vi "XY Galvo Generator Underscan.v2.Filter.vi"(3 "Microscope Settings in":T1={"Mode"=enum."X", "Slit"={"Scanning Mode"=0.0, "Slit Width /%"=0.0}, "Colour Channel"=enum."3", "Colour"=[], "Focus Offset /um"=0.0, "Exposure/ms"=0.0, "Piezo Position /um"=0.0, "ROI"={"X"={"Start /px"=0.0, "Step /px"=0.0, "Range /px"=0.0}, "Y"={"Start /px"=0.0, "Step /px"=0.0, "Range /px"=0.0}, "Z "={"Start /um"=0.0, "Step/um"=0.0, "Range /um"=0.0}, "T "={"Start /s"=0.0, "Step /s"=1.0, "Range /s"=100.0}}, "Samples per millisecond"=0.0, "Relax/ms"=0.0, "Readout Direction"=0.0, "Trigger Source"=0.0, "Camera Delay /ms"=0.0, "Under Scan /ms"=0.0, "Slit Delay"=100.0, "Waveforms"={"Analogue Out"=[{"t0"=timestamp(0 s since 1904-01-01), "dt"=1.0, "Y"=[]}, {"t0"=timestamp(0 s since 1904-01-01), "dt"=1.0, "Y"=[]}, {"t0"=timestamp(0 s since 1904-01-01), "dt"=1.0, "Y"=[]}], "Digital Out"=[{"t0"=timestamp(0 s since 1904-01-01), "dt"=0.0, "Y"={"transitions"=[], "data"=[]}}, {"t0"=timestamp(0 s since 1904-01-01), "dt"=0.0, "Y"={"transitions"=[], "data"=[]}}, {"t0"=timestamp(0 s since 1904-01-01), "dt"=0.0, "Y"={"transitions"=[], "data"=[]}}]}} {"Focus Offset /um" min=0.0 max=10.0 step=0.05 scale=-2.0..2.0 scale format="%.2f"; "ROI"."T"."Range /s" min=0.0 max=10.0 step=0.05; "ROI"."T"."Step /s" min=0.0 max=10.0 step=0.05; "ROI"."T"."Start /s" min=0.0 max=10.0 step=0.05; "ROI"."X"."Range /px" min=0.0 max=10.0 step=0.05; "ROI"."X"."Step /px" min=0.0 max=10.0 step=0.05; "ROI"."X"."Start /px" min=0.0 max=10.0 step=0.05; "ROI"."Y"."Range /px" min=0.0 max=10.0 step=0.05; "ROI"."Y"."Step /px" min=0.0 max=10.0 step=0.05; "ROI"."Y"."Start /px" min=0.0 max=10.0 step=0.05; "ROI"."Z"."Range /um" min=0.0 max=10.0 step=0.05; "ROI"."Z"."Step/um" min=0.0 max=10.0 step=0.05; "ROI"."Z"."Start /um" min=0.0 max=10.0 step=0.05; "Colour"."Colour"."Filter" items=["Empty"=1, ""=2, ""=3, "561"=4, ""=5, "488"=6]; "Camera Delay /ms" min=0.0 max=10.0 step=0.05; "Trigger Source" items=["Internal"=1.0, "External"=2.0]; "Readout Direction" items=["Internal"=1.0, "External"=2.0]; "Slit"."Scanning Mode" items=["Full Frame"=1.0, "Slit Scanning"=12.0]; "Piezo Position /um" min=0.0 max=10.0 step=0.05; "Exposure/ms" min=0.0 max=10.0 step=0.05; "Samples per millisecond" min=1.0 max=2.0 step=1.0}) -> (0 "Piezo":dbl[](graph))   [LabVIEW 2016]
uses:
  controls/Microscope Settings.ctl
  controls/ColourCalibration.ctl
panel:
  in  "Filter Voltage":dbl
  out "Signal":dbl[](array[numeric])
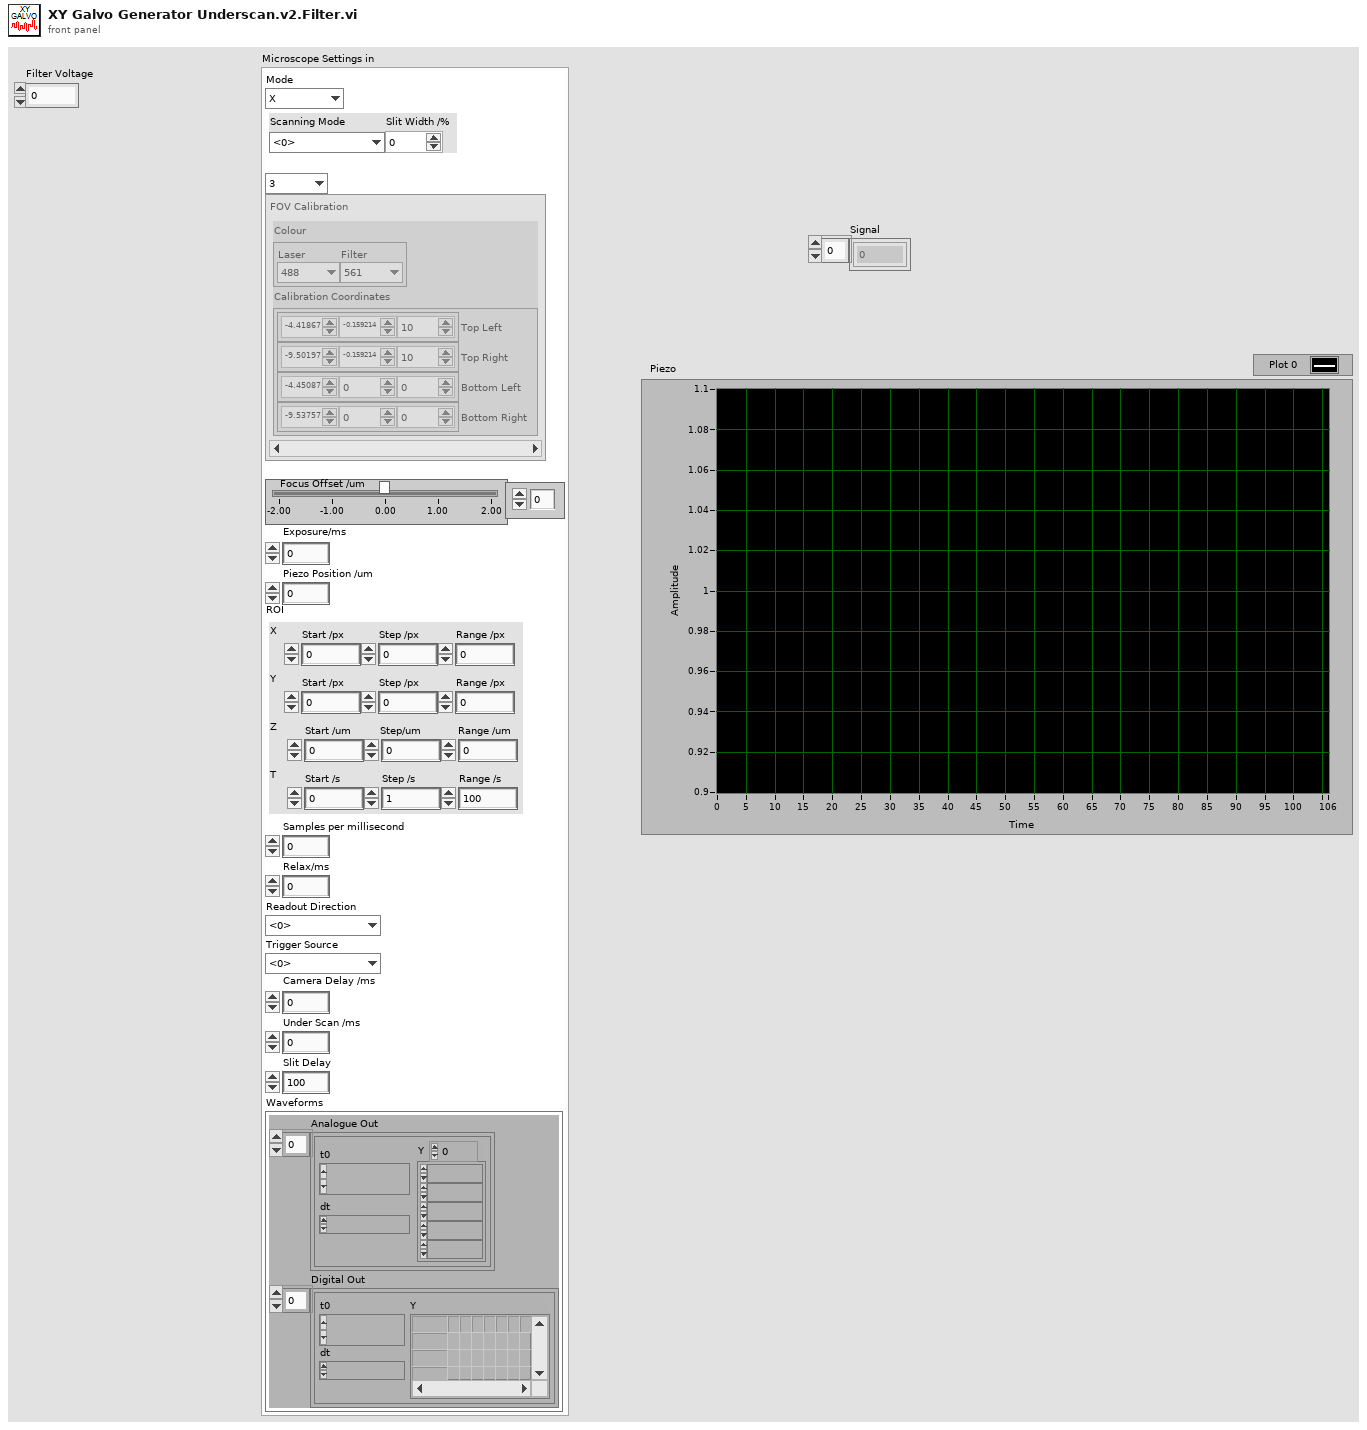
[diagram p1: front panel]
types:
  T1 = typedef "Microscope Settings.ctl" = cluster{"Mode":enum16{"Brightfield", "X", "XY", "XYZ", "XYC", "XYCT", "XYZT", "XYZC", "Tweezers", "Virus"}, "Slit":cluster{"Scanning Mode":dbl, "Slit Width /%":dbl}, "Colour Channel":enum16{"1", "2", "3", "4", "5"}, "Colour":T2, "Focus Offset /um":dbl, "Exposure/ms":dbl, "Piezo Position /um":dbl, "ROI":cluster{"X":cluster{"Start /px":dbl, "Step /px":dbl, "Range /px":dbl}, "Y":cluster{"Start /px":dbl, "Step /px":dbl, "Range /px":dbl}, "Z ":cluster{"Start /um":dbl, "Step/um":dbl, "Range /um":dbl}, "T ":cluster{"Start /s":dbl, "Step /s":dbl, "Range /s":dbl}}, "Samples per millisecond":dbl, "Relax/ms":dbl, "Readout Direction":dbl, "Trigger Source":dbl, "Camera Delay /ms":dbl, "Under Scan /ms":dbl, "Slit Delay":dbl, "Waveforms":cluster{"Analogue Out":waveform(dbl)[], "Digital Out":digitalwaveform[]}}
  T2 = typedef "ColourCalibration.ctl" = cluster{"Colour":cluster{"Laser":enum16{"Brightfield", "445", "488", "561", "647"}, "Filter":u16}, "Calibration Coordinates":cluster{"Top Left":dbl[], "Top Right":dbl[], "Bottom Left":dbl[], "Bottom Right":dbl[]}}[]
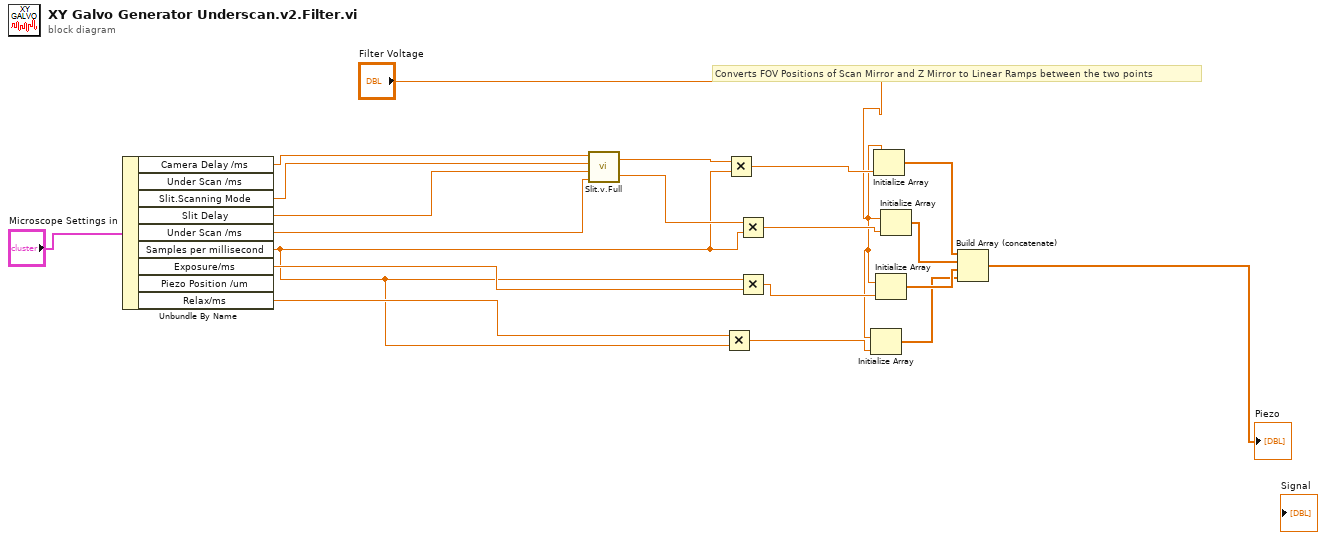
[diagram p0: block diagram]
diagram:
  # "Converts FOV Positions of Scan Mirror and Z Mirror to Linear Ramps between the two points"
  n1 = Unbundle By Name("Microscope Settings in") -> ("Camera Delay /ms"=w16:dbl, "Slit.Scanning Mode"=w17:dbl, "Slit Delay"=w18:dbl, "Under Scan /ms"=w19:dbl, "Samples per millisecond"=w11:dbl, "Exposure/ms"=w15:dbl, "Relax/ms"=w14:dbl)  [unwired: 2 out]
  n2 = call "Slit.v.Full.vi"("Under Scan /ms"=w19, "Slit Delay"=w18, "Scanning Mode"=w17, "Camera Delay /ms"=w16) -> ("Prexposure /ms"=w12:dbl, "Underscan /ms"=w13:dbl)
  n3 = Multiply(x=w14, y=w11) -> (x*y=w7:dbl)
  n4 = Multiply(x=w13, y=w11) -> (x*y=w10:dbl)
  n5 = Multiply(x=w12, y=w11) -> (x*y=w9:dbl)
  n6 = Multiply(x=w11, y=w15) -> (x*y=w8:dbl)
  n7 = Initialize Array("Filter Voltage", w7) -> (w2:dbl[])
  n8 = Initialize Array("Filter Voltage", w10) -> (w5:dbl[])
  n9 = Initialize Array("Filter Voltage", w8) -> (w3:dbl[])
  n10 = Initialize Array("Filter Voltage", w9) -> (w4:dbl[])
  n11 = Build Array (concatenate)(w5, w4, w3, w2) -> (→"Piezo":dbl[])
